vi "Simon.vi"() -> ()   [LabVIEW 2021]
uses:
  <vilib>/Platform/TimedLoop/XDataNode/timing_clust.ctl
  <vilib>/Platform/TimedLoop/XDataNode/nitl_modes.ctl
  <vilib>/Platform/TimedLoop/XDataNode/wakeup.ctl
  <vilib>/platform/TimedLoop/XDataNode/XDataNode.xnode
  <vilib>/Platform/TimedLoop/XDataNode/XDNodeRunTimeDep.lvlib
panel:
  out "Try Again":bool
  out "Game Over":bool
  out "Streak":i32
  in  "Blue":bool
  in  "Green":bool
  in  "Yellow":bool
  in  "Red":bool
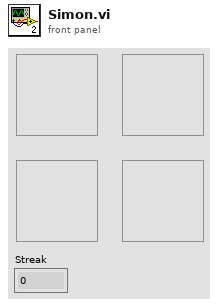
[diagram p1: front panel]
types:
  T1 = cluster{"Sequence":i32[], "Current Index To Check":i32}
  T2 = enum16{"Link Start", "Add Round", "Show Rounds", "Wait", "Validate", "Victory", "Defeat", "Link End"}
  T3 = typedef "XDNodeRunTimeDep.lvlib/timing_clust.ctl" = cluster{"Expected End [f-1]":u64, "Actual End [f-1]":u64, "Finished Late? [f-1]":bool, "Expected End [i-1]":u64, "Actual End [i-1]":u64, "Finished Late? [i-1]":bool, "Expected Start [i]":u64, "Actual Start [i]":u64, "Expected Start [f]":u64, "Actual Start [f]":u64, "Source Name":string, "Structure Name":string, "Period":i64, "Deadline":i64, "Offset":i64, "Start":i64, "Priority":i32, "Timeout":i32, "Mode":T4, "Wakeup Reason":T5, "Error":errorcluster, "Source Type":string, "Secondary Source Type":string, "Global End Time":u64, "Global Start Time":u64, "Frame Duration":u64, "Iteration Duration":u64, "Assigned CPU":i32, "I/O Scan Engine Mode":u32}
  T4 = typedef "XDNodeRunTimeDep.lvlib/nitl_modes.ctl" = enum32{"No Change", "Process missed periods, maintain original phase", "Discard missed periods, maintain original phase", "Process missed periods, ignore original phase", "Discard missed periods, ignore original phase"}
  T5 = typedef "XDNodeRunTimeDep.lvlib/wakeup.ctl" = enum32{"Normal", "Aborted", "Asynchronous wakeup", "Timing source error", "Timed loop error", "Timeout"}
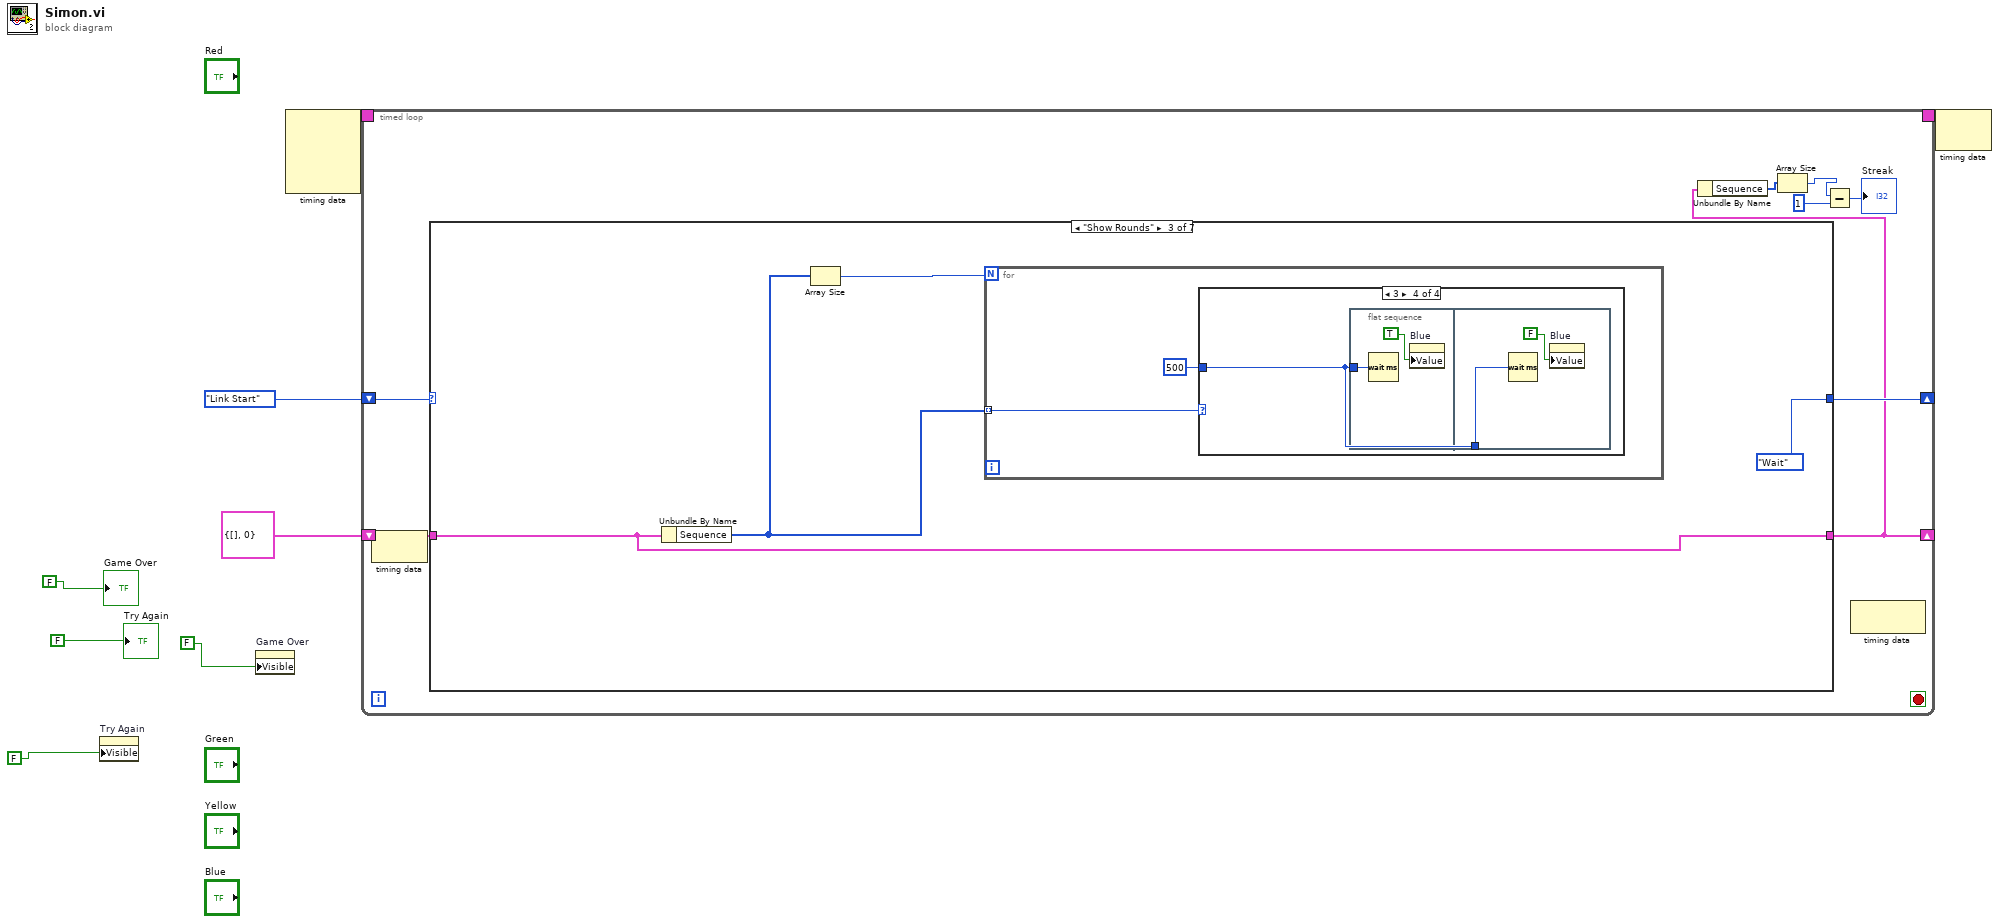
[diagram p0: block diagram]
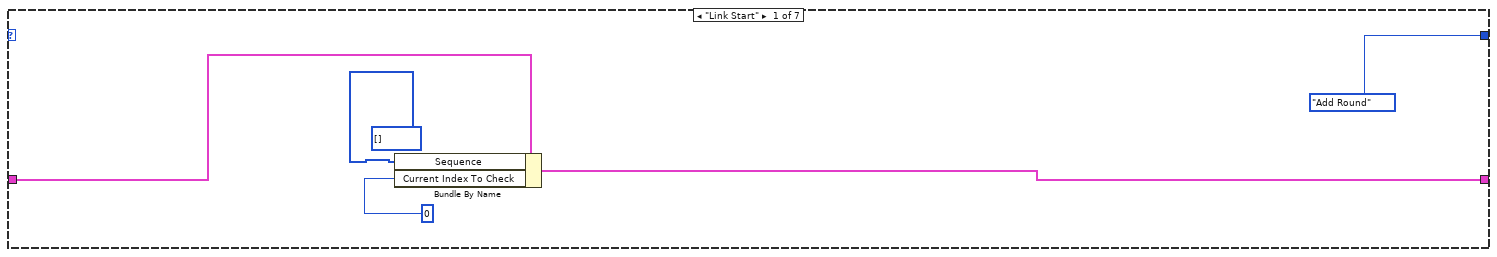
[diagram p2: hidden frame]
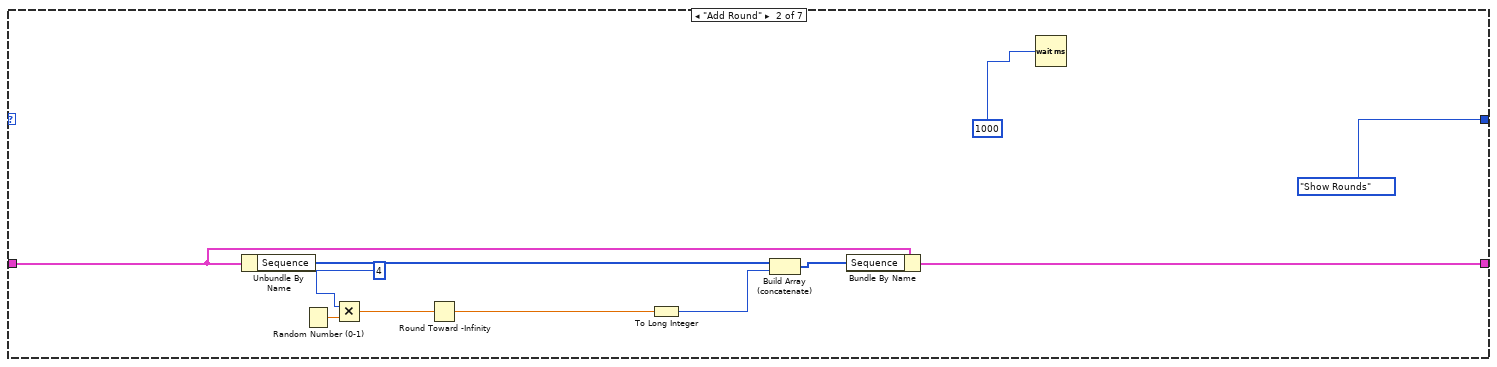
[diagram p3: hidden frame]
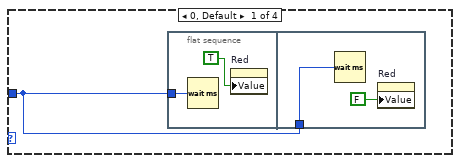
[diagram p4: hidden frame]
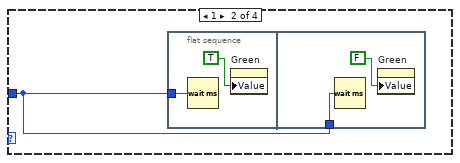
[diagram p5: hidden frame]
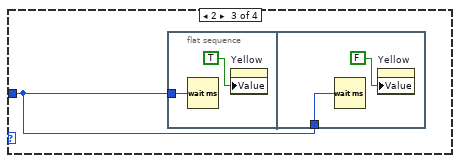
[diagram p6: hidden frame]
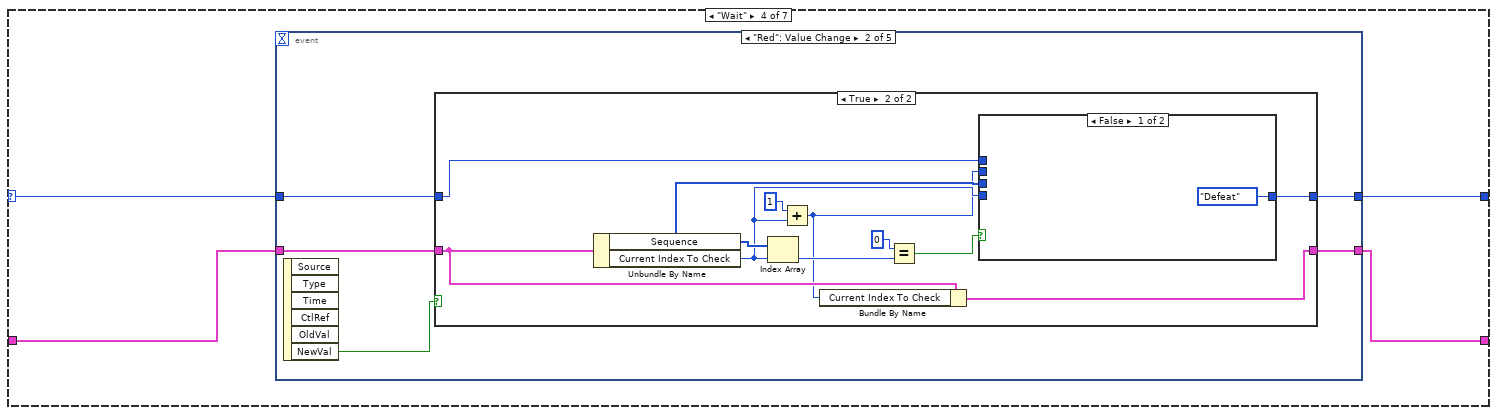
[diagram p7: hidden frame]
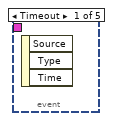
[diagram p8: hidden frame]
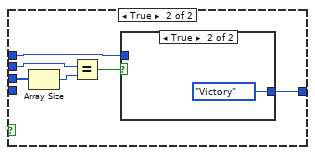
[diagram p10: hidden frame]
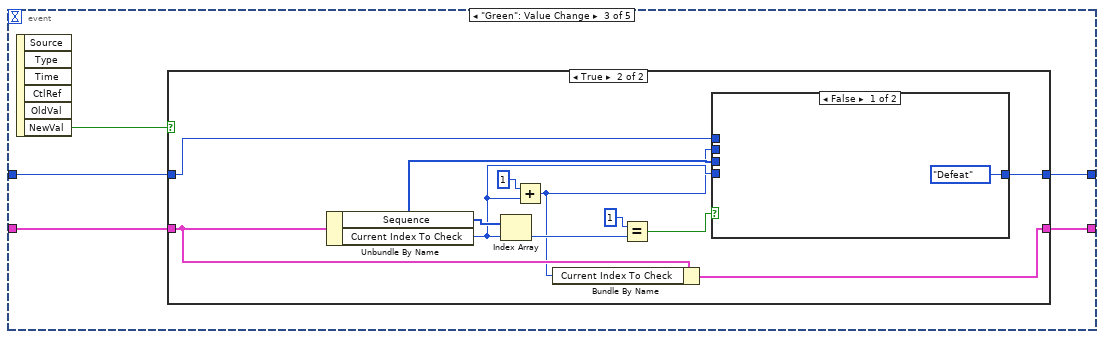
[diagram p12: hidden frame]
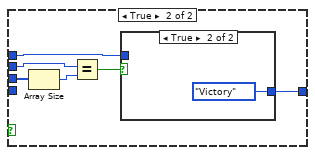
[diagram p14: hidden frame]
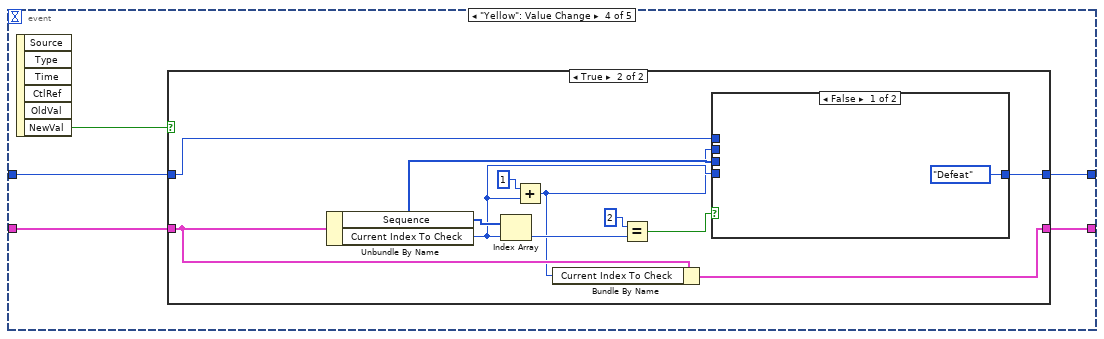
[diagram p16: hidden frame]
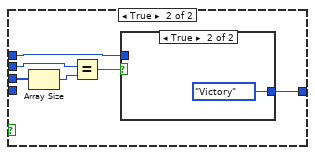
[diagram p18: hidden frame]
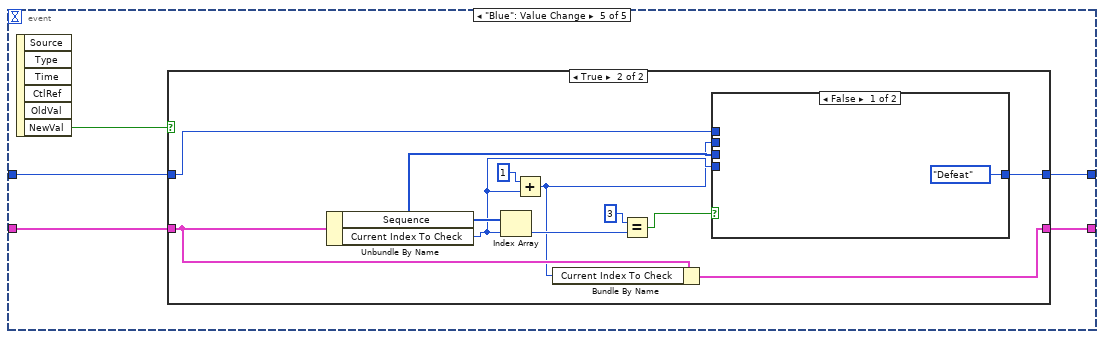
[diagram p20: hidden frame]
diagram:
  n1 = property on="Try Again" class="Bool (strict)"("Visible"=FALSE) -> ()  [unwired: 2 in, 2 out]
  n2 = property on="Game Over" class="Bool (strict)"("Visible"=FALSE) -> ()  [unwired: 2 in, 2 out]
  n3 = node-c288() -> (w7:T3)  [unwired: 4 in]
  n4 = timed-loop {
    shift-right: [w15] -> _
    shift-left: T2."Link Start" -> [w16]
    timing: w7 -> [_]
    timing-out: [_] -> w6
    shift-right: [w12] -> _
    shift-left: T1 {"Sequence"=[], "Current Index To Check"=0} -> [w14]
    stop <- _ stop-if-true
    n5 = node-c288() -> ()  [unwired: 1 in, 1 out]
    n6 = case shown="\"Show Rounds\"" w16 {
      selector: w16 -> [_ _ _ w61 _ _ w187]
      tunnel: [w22 w28 w38 w63 w175 w178 w188] -> w12
      tunnel: w14 -> [w23 w30 w38 w64 w174 w178 w188]
      tunnel: [T2."Add Round" T2."Show Rounds" T2."Wait" w62 T2."Add Round" T2."Link Start" w187] -> w15
      frame "Link Start" {
        n7 = Bundle By Name(cluster=w23, "Sequence"=i32[] [], "Current Index To Check"=0) -> (w22:T1)
      }
      frame "Add Round" {
        n8 = Unbundle By Name(w30) -> ("Sequence"=w31:i32[])
        n9 = Random Number (0-1)() -> (number: 0 to 1=w34:dbl)
        n10 = Multiply(x=4, y=w34) -> (x*y=w32:dbl)
        n11 = Round Toward -Infinity(1:w32) -> (0:w27:dbl)
        n12 = To Long Integer(number=w27) -> (32bit integer=w26:i32)
        n13 = Build Array (concatenate)(w31, w26) -> (w29:i32[])
        n14 = Bundle By Name(cluster=w30, "Sequence"=w29) -> (w28:T1)
        n15 = Wait (ms)(milliseconds to wait=1000) -> ()  [unwired: 1 out]
      }
      frame "Show Rounds" {
        n16 = Unbundle By Name(w38) -> ("Sequence"=w37:i32[])
        n17 = Array Size(array=w37) -> (size(s)=w36:i32)
        n18 = for {
          N: w36 -> [_]
          tunnel: w37 -> [w40] mode=indexing
          n19 = case shown="3" w40 {
            tunnel: 500 -> [w41 w46 w51 w56]
            frame 0, Default {
              n20 = flat-sequence {
                tunnel: w41 -> [w43]
                tunnel: w41 -> [w44]
                frame #0 {
                  n21 = Wait (ms)(milliseconds to wait=w43) -> ()  [unwired: 1 out]
                  n22 = property on="Red" class="Bool (strict)"("Value"=TRUE) -> ()  [unwired: 2 in, 2 out]
                }
                frame #1 {
                  n23 = Wait (ms)(milliseconds to wait=w44) -> ()  [unwired: 1 out]
                  n24 = property on="Red" class="Bool (strict)"("Value"=FALSE) -> ()  [unwired: 2 in, 2 out]
                }
              }
            }
            frame 1 {
              n25 = flat-sequence {
                tunnel: w46 -> [w48]
                tunnel: w46 -> [w49]
                frame #0 {
                  n26 = Wait (ms)(milliseconds to wait=w48) -> ()  [unwired: 1 out]
                  n27 = property on="Green" class="Bool (strict)"("Value"=TRUE) -> ()  [unwired: 2 in, 2 out]
                }
                frame #1 {
                  n28 = Wait (ms)(milliseconds to wait=w49) -> ()  [unwired: 1 out]
                  n29 = property on="Green" class="Bool (strict)"("Value"=FALSE) -> ()  [unwired: 2 in, 2 out]
                }
              }
            }
            frame 2 {
              n30 = flat-sequence {
                tunnel: w51 -> [w53]
                tunnel: w51 -> [w54]
                frame #0 {
                  n31 = Wait (ms)(milliseconds to wait=w53) -> ()  [unwired: 1 out]
                  n32 = property on="Yellow" class="Bool (strict)"("Value"=TRUE) -> ()  [unwired: 2 in, 2 out]
                }
                frame #1 {
                  n33 = Wait (ms)(milliseconds to wait=w54) -> ()  [unwired: 1 out]
                  n34 = property on="Yellow" class="Bool (strict)"("Value"=FALSE) -> ()  [unwired: 2 in, 2 out]
                }
              }
            }
            frame 3 {
              n35 = flat-sequence {
                tunnel: w56 -> [w58]
                tunnel: w56 -> [w59]
                frame #0 {
                  n36 = Wait (ms)(milliseconds to wait=w58) -> ()  [unwired: 1 out]
                  n37 = property on="Blue" class="Bool (strict)"("Value"=TRUE) -> ()  [unwired: 2 in, 2 out]
                }
                frame #1 {
                  n38 = Wait (ms)(milliseconds to wait=w59) -> ()  [unwired: 1 out]
                  n39 = property on="Blue" class="Bool (strict)"("Value"=FALSE) -> ()  [unwired: 2 in, 2 out]
                }
              }
            }
          }
        }
      }
      frame "Wait" {
        n40 = event shown="[1] \"Red\": Value Change" {
          selector: _ -> [_ _ _ _ _]
          dyn-events: _ -> [_ _ _ _ _]
          timeout: _ -> [_ _ _ _ _]
          tunnel: w64 -> [_ w68 w95 w122 w149]
          tunnel: [_ w67 w94 w121 w148] -> w63
          tunnel: [_ w66 w93 w120 w147] -> w62
          tunnel: w61 -> [_ w65 w92 w119 w146]
          event Timeout {
            n41 = event-data() -> ()  [unwired: 1 in, 3 out]
          }
          event "Red": Value Change {
            n42 = event-data() -> ("NewVal"=w69:bool)  [unwired: 1 in, 5 out]
            n43 = case shown="True" w69 {
              tunnel: w68 -> [w71 w78]
              tunnel: [w71 w79] -> w67
              tunnel: [w70 w76] -> w66
              tunnel: w65 -> [w70 w72]
              frame False {
              }
              frame True {
                n44 = Unbundle By Name(w78) -> ("Sequence"=w77:i32[], "Current Index To Check"=w74:i32)
                n45 = Index Array(array=w77, index=w74) -> (element=w82:i32)
                n46 = Add(x=1, y=w74) -> (x+y=w73:i32)
                n47 = Bundle By Name(cluster=w78, "Current Index To Check"=w73) -> (w79:T1)
                n48 = Equal?(x=0, y=w82) -> (x = y?=w80:bool)
                n49 = case shown="False" w80 {
                  tunnel: w74 -> [_ _]
                  tunnel: w77 -> [_ w89]
                  tunnel: [T2."Defeat" w86] -> w76
                  tunnel: w73 -> [_ w85]
                  tunnel: w72 -> [_ w84]
                  frame False {
                  }
                  frame True {
                    n50 = Array Size(array=w89) -> (size(s)=w88:i32)
                    n51 = Equal?(x=w85, y=w88) -> (x = y?=w87:bool)
                    n52 = case shown="True" w87 {
                      tunnel: [w90 T2."Victory"] -> w86
                      tunnel: w84 -> [w90 _]
                      frame False {
                      }
                      frame True {
                      }
                    }
                  }
                }
              }
            }
          }
          event "Green": Value Change {
            n53 = event-data() -> ("NewVal"=w96:bool)  [unwired: 1 in, 5 out]
            n54 = case shown="True" w96 {
              tunnel: w95 -> [w98 w105]
              tunnel: [w98 w106] -> w94
              tunnel: [w97 w103] -> w93
              tunnel: w92 -> [w97 w99]
              frame False {
              }
              frame True {
                n55 = Unbundle By Name(w105) -> ("Sequence"=w104:i32[], "Current Index To Check"=w101:i32)
                n56 = Index Array(array=w104, index=w101) -> (element=w109:i32)
                n57 = Add(x=1, y=w101) -> (x+y=w100:i32)
                n58 = Bundle By Name(cluster=w105, "Current Index To Check"=w100) -> (w106:T1)
                n59 = Equal?(x=1, y=w109) -> (x = y?=w107:bool)
                n60 = case shown="False" w107 {
                  tunnel: w101 -> [_ _]
                  tunnel: w104 -> [_ w116]
                  tunnel: [T2."Defeat" w113] -> w103
                  tunnel: w100 -> [_ w112]
                  tunnel: w99 -> [_ w111]
                  frame False {
                  }
                  frame True {
                    n61 = Array Size(array=w116) -> (size(s)=w115:i32)
                    n62 = Equal?(x=w112, y=w115) -> (x = y?=w114:bool)
                    n63 = case shown="True" w114 {
                      tunnel: [w117 T2."Victory"] -> w113
                      tunnel: w111 -> [w117 _]
                      frame False {
                      }
                      frame True {
                      }
                    }
                  }
                }
              }
            }
          }
          event "Yellow": Value Change {
            n64 = event-data() -> ("NewVal"=w123:bool)  [unwired: 1 in, 5 out]
            n65 = case shown="True" w123 {
              tunnel: w122 -> [w125 w132]
              tunnel: [w125 w133] -> w121
              tunnel: [w124 w130] -> w120
              tunnel: w119 -> [w124 w126]
              frame False {
              }
              frame True {
                n66 = Unbundle By Name(w132) -> ("Sequence"=w131:i32[], "Current Index To Check"=w128:i32)
                n67 = Index Array(array=w131, index=w128) -> (element=w136:i32)
                n68 = Add(x=1, y=w128) -> (x+y=w127:i32)
                n69 = Bundle By Name(cluster=w132, "Current Index To Check"=w127) -> (w133:T1)
                n70 = Equal?(x=2, y=w136) -> (x = y?=w134:bool)
                n71 = case shown="False" w134 {
                  tunnel: w128 -> [_ _]
                  tunnel: w131 -> [_ w143]
                  tunnel: [T2."Defeat" w140] -> w130
                  tunnel: w127 -> [_ w139]
                  tunnel: w126 -> [_ w138]
                  frame False {
                  }
                  frame True {
                    n72 = Array Size(array=w143) -> (size(s)=w142:i32)
                    n73 = Equal?(x=w139, y=w142) -> (x = y?=w141:bool)
                    n74 = case shown="True" w141 {
                      tunnel: [w144 T2."Victory"] -> w140
                      tunnel: w138 -> [w144 _]
                      frame False {
                      }
                      frame True {
                      }
                    }
                  }
                }
              }
            }
          }
          event "Blue": Value Change {
            n75 = event-data() -> ("NewVal"=w150:bool)  [unwired: 1 in, 5 out]
            n76 = case shown="True" w150 {
              tunnel: w149 -> [w152 w159]
              tunnel: [w152 w160] -> w148
              tunnel: [w151 w157] -> w147
              tunnel: w146 -> [w151 w153]
              frame False {
              }
              frame True {
                n77 = Unbundle By Name(w159) -> ("Sequence"=w158:i32[], "Current Index To Check"=w155:i32)
                n78 = Index Array(array=w158, index=w155) -> (element=w163:i32)
                n79 = Add(x=1, y=w155) -> (x+y=w154:i32)
                n80 = Bundle By Name(cluster=w159, "Current Index To Check"=w154) -> (w160:T1)
                n81 = Equal?(x=3, y=w163) -> (x = y?=w161:bool)
                n82 = case shown="False" w161 {
                  tunnel: w155 -> [_ _]
                  tunnel: w158 -> [_ w170]
                  tunnel: [T2."Defeat" w167] -> w157
                  tunnel: w154 -> [_ w166]
                  tunnel: w153 -> [_ w165]
                  frame False {
                  }
                  frame True {
                    n83 = Array Size(array=w170) -> (size(s)=w169:i32)
                    n84 = Equal?(x=w166, y=w169) -> (x = y?=w168:bool)
                    n85 = case shown="True" w168 {
                      tunnel: [w171 T2."Victory"] -> w167
                      tunnel: w165 -> [w171 _]
                      frame False {
                      }
                      frame True {
                      }
                    }
                  }
                }
              }
            }
          }
        }
      }
      frame "Victory" {
        n86 = Bundle By Name(cluster=w174, "Current Index To Check"=0) -> (w175:T1)
      }
      frame "Defeat" {
        n87 = flat-sequence {
          frame #0 {
            n88 = for {
              N: 3 -> [_]
              n89 = flat-sequence {
                frame #0 {
                  n90 = property on="Game Over" class="Bool (strict)"("Visible"=TRUE) -> ()  [unwired: 2 in, 2 out]
                  n91 = Wait (ms)(milliseconds to wait=500) -> ()  [unwired: 1 out]
                }
                frame #1 {
                  n92 = property on="Game Over" class="Bool (strict)"("Visible"=FALSE) -> ()  [unwired: 2 in, 2 out]
                  n93 = Wait (ms)(milliseconds to wait=500) -> ()  [unwired: 1 out]
                }
              }
            }
          }
          frame #1 {
            n94 = property on="Try Again" class="Bool (strict)"("Visible"=TRUE) -> ()  [unwired: 2 in, 2 out]
            n95 = Wait (ms)(milliseconds to wait=2000) -> ()  [unwired: 1 out]
          }
          frame #2 {
            n96 = property on="Try Again" class="Bool (strict)"("Visible"=FALSE) -> ()  [unwired: 2 in, 2 out]
          }
        }
      }
      frame "Link End", Default {
      }
    }
    n97 = Unbundle By Name(w12) -> ("Sequence"=w13:i32[])
    n98 = Array Size(array=w13) -> (size(s)=w11:i32)
    n99 = Subtract(x=w11, y=1) -> (x-y=→"Streak":i32)
    n100 = node-c288() -> ()  [unwired: 1 in, 1 out]
  }
  n101 = node-c288(w6) -> ()  [unwired: 1 out]
  "Game Over" <- FALSE
  "Try Again" <- FALSE
